vi "Message.vi"() -> (0 "Reason 2":string, 3 "Cancelled?":bool)   [LabVIEW 2010]
doc: "Use this template to create a dialog box. This template polls the state of the buttons on the front panel and does not use events. Use the Dialog Using Events template (not available in Base package) to create a dialog box with event handling."
panel:
  in  "Reason":string caption="Опишите причину внеочередной записи"
  in  "Cancel":bool
  in  "OK":bool
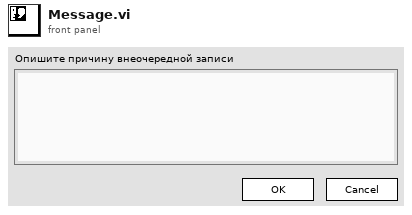
[diagram p1: front panel]
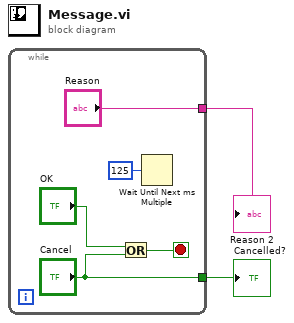
[diagram p0: block diagram]
diagram:
  n1 = while {
    tunnel: ["Cancel"] -> w2
    tunnel: ["Reason"] -> w1
    stop <- w6 stop-if-true
    n2 = Or(x="OK", y="Cancel") -> (x .or. y?=w6:bool)
    n3 = Wait Until Next ms Multiple(millisecond multiple=u32 125) -> ()  [unwired: 1 out]
  }
  "Cancelled?" <- w2
  "Reason 2" <- w1
